vi "Dispose Ref.vi"(8 "error in (no error)":errorcluster caption="错误输入（无错误）", 11 "StatusStripClass 输入":refnum<class "StatusStripClass.lvclass"> caption="DNL_LabVIEW Object in") -> (0 "error out":errorcluster caption="错误输出")   [LabVIEW 2013, in "StatusStripClass.lvclass"]
uses:
  StatusStripClass.lvclass
  StatusStripClass.lvclass/StatusStripClass.ctl
  System.Windows.Forms
panel:
  out "StatusStripClass 输出":refnum<class "StatusStripClass.lvclass"> caption="DNL_LabVIEW Object out"
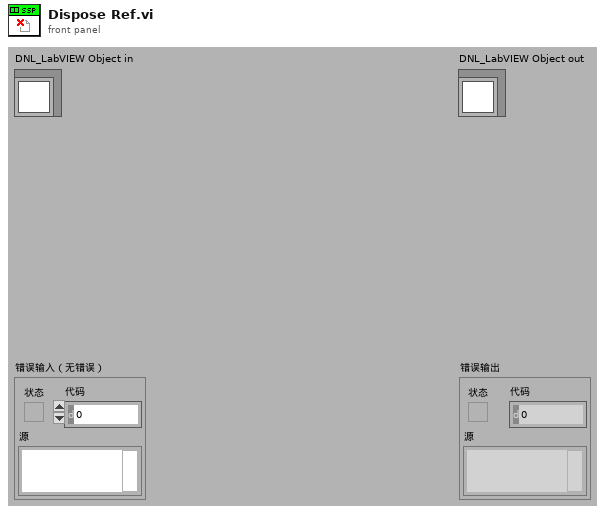
[diagram p1: front panel]
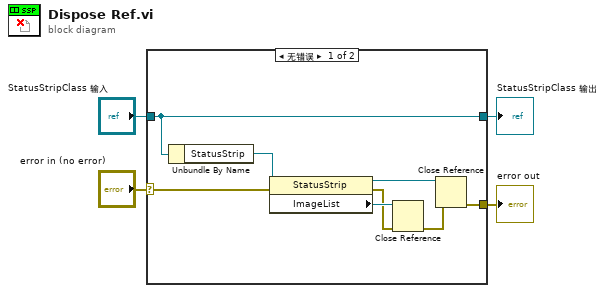
[diagram p0: block diagram]
diagram:
  n1 = case shown="无错误" "error in (no error)" {
    selector: "error in (no error)" -> [w9 w14]
    tunnel: [w7 w14] -> w3
    tunnel: [w12 w13] -> w1
    tunnel: "StatusStripClass 输入" -> [w12 w13]
    frame No Error {
      n2 = Unbundle By Name(w12) -> ("StatusStrip"=w11:refnum<k24>)
      n3 = property class="StatusStrip"(reference=w11, error in=w9) -> (reference out=w5:refnum<k24>, error out=w6:errorcluster, "ImageList"=w10:refnum<k24>)
      n4 = Close Reference(reference=w10, error in (no error)=w6) -> (error out=w8:errorcluster)
      n5 = Close Reference(reference=w5, error in (no error)=w8) -> (error out=w7:errorcluster)
    }
    frame Error {
    }
  }
  "error out" <- w3
  "StatusStripClass 输出" <- w1
